vi "setValue.vi"(8 "error in (no error)":errorcluster, 10 "Value":refnum<class "tBSONElement.lvclass">[](array[class]), 11 "tBSONArray in":refnum<class "tBSONArray.lvclass">) -> (0 "error out":errorcluster, 3 "tBSONArray out":refnum<class "tBSONArray.lvclass">)   [LabVIEW 2013, in "BSON.lvlib" / "tBSONArray.lvclass"]
uses:
  tBSONArray.lvclass
  tBSONElement/tBSONElement.lvclass
  tBSONArray.lvclass/tBSONArray.ctl
  tBSONElement/setName.vi
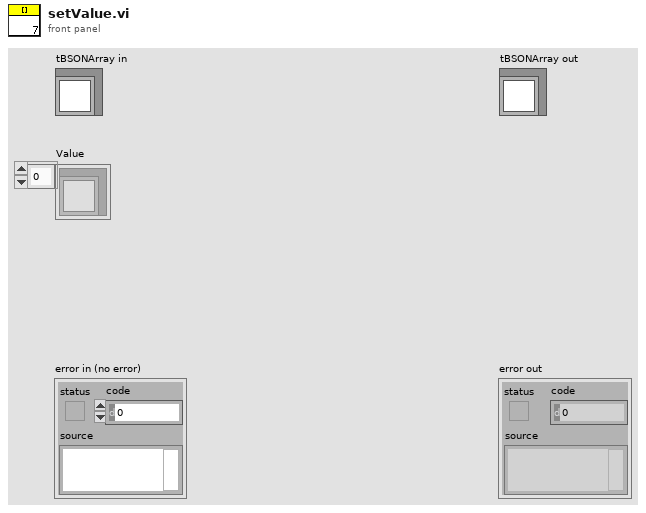
[diagram p1: front panel]
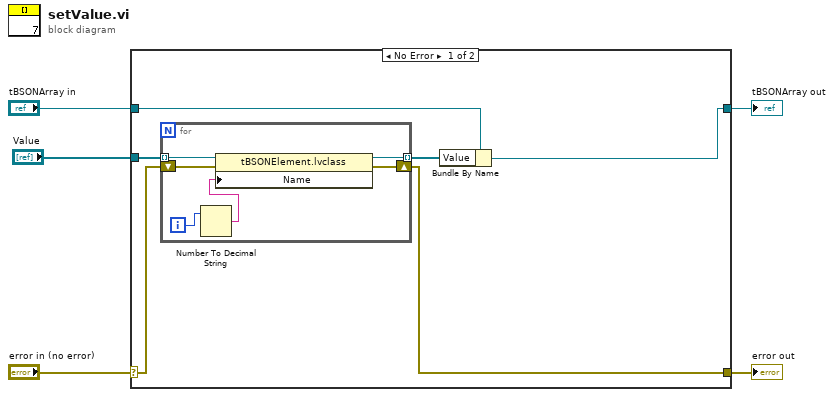
[diagram p0: block diagram]
diagram:
  n1 = case shown="No Error" "error in (no error)" {
    selector: "error in (no error)" -> [w7 w19]
    tunnel: [w6 w19] -> w4
    tunnel: [w10 w18] -> w2
    tunnel: "tBSONArray in" -> [w11 w18]
    tunnel: "Value" -> [w9 _]
    frame No Error {
      n2 = for {
        tunnel: w9 -> [w17] mode=indexing
        tunnel: [w15] -> w8 mode=indexing
        shift-right: [w14] -> w6
        shift-left: w7 -> [w16]
        i -> [w13]
        n3 = Number To Decimal String(number=w13) -> (decimal integer string=w12:string)  [unwired: 1 in]
        n4 = property class="tBSONElement.lvclass"(reference=w17, error in=w16, "Name"=w12) -> (reference out=w15:refnum<class "tBSONElement.lvclass">, error out=w14:errorcluster)
      }
      n5 = Bundle By Name(cluster=w11, "Value"=w8) -> (w10:refnum<class "tBSONArray.lvclass">)
    }
    frame Error {
    }
  }
  "error out" <- w4
  "tBSONArray out" <- w2
